vi "background.vi"(10 "Enum":enum16{"clear", "read", "write"}(ring)=enum."write", 11 "backgroundImageIn":i32[][](array[numeric])) -> (3 "backgroundImageOut":i32[][](array[numeric]))   [LabVIEW 2016]
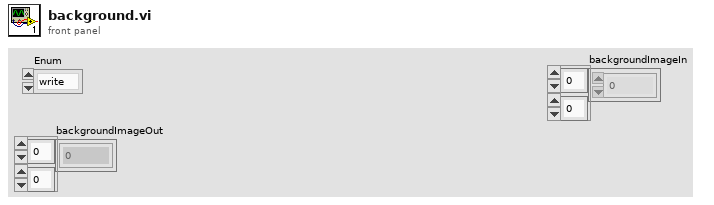
[diagram p1: front panel]
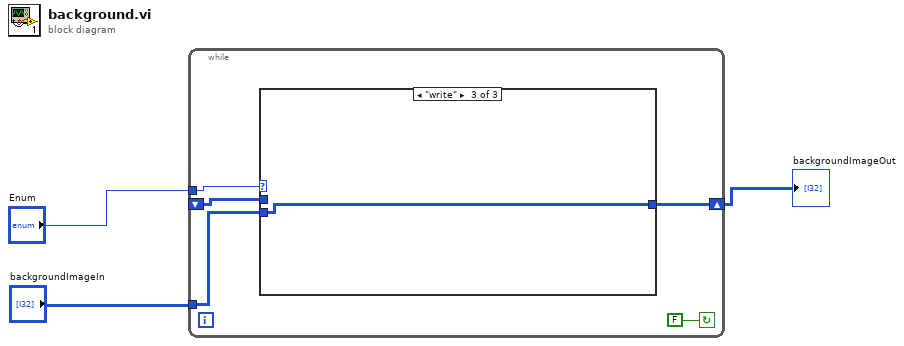
[diagram p0: block diagram]
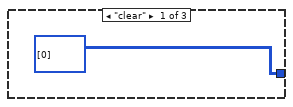
[diagram p2: hidden frame]
diagram:
  n1 = while {
    tunnel: "Enum" -> [w7]
    shift-right: [w6] -> w2
    shift-left: _ -> [w4]
    tunnel: "backgroundImageIn" -> [w5]
    stop <- FALSE continue-if-true
    n2 = case shown="\"write\"" w7 {
      tunnel: w5 -> [_ _ w11]
      tunnel: [i32[][] [[0]] ("imageCube") w10 w11] -> w6
      tunnel: w4 -> [_ w10 _]
      frame "clear" {
      }
      frame "read", Default {
      }
      frame "write" {
      }
    }
  }
  "backgroundImageOut" <- w2
